vi "Deposition-needed.vi"(8 "error in (no error)":errorcluster, 11 "Object ref in":T1) -> (0 "error out":errorcluster, 1 "Deposit?":bool, 3 "Object ref out":T1)   [LabVIEW 2013, in "SLMControl.lvlib" / "SC-Main.lvclass"]
uses:
  SC-Main.lvclass
  Object-reference.ctl
  SC-Main.lvclass/SC-Main.ctl
  Read Deposition files.vi
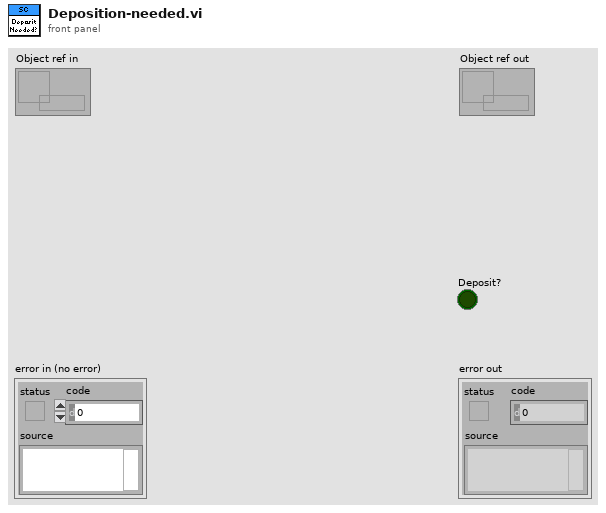
[diagram p1: front panel]
types:
  T1 = typedef "SLMControl.lvlib/SC-Main.lvclass/Object-reference.ctl" = refnum<data-value>
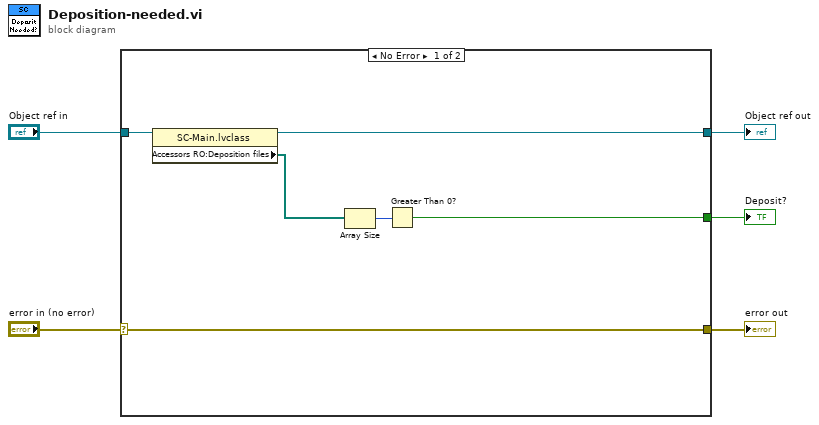
[diagram p0: block diagram]
diagram:
  n1 = case shown="No Error" "error in (no error)" {
    selector: "error in (no error)" -> [w11 w13]
    tunnel: [w11 w13] -> w4
    tunnel: [w9 w12] -> w2
    tunnel: "Object ref in" -> [w10 w12]
    tunnel: [w6 _] -> w1
    frame No Error {
      n2 = property class="SC-Main.lvclass"(reference=w10) -> (reference out=w9:T1, "Accessors RO:Deposition files"=w7:path[])  [unwired: 1 in, 1 out]
      n3 = Array Size(array=w7) -> (size(s)=w8:i32)
      n4 = Greater Than 0?(x=w8) -> (x > 0?=w6:bool)
    }
    frame Error {
    }
  }
  "error out" <- w4
  "Object ref out" <- w2
  "Deposit?" <- w1
